vi "Read Interval.vi"(8 "error in (no error)":errorcluster, 11 "CS++PVMonitor in":refnum<class "CS++PVMonitor.lvclass">) -> (0 "error out":errorcluster, 2 "Interval":dbl[unit], 3 "CS++PVMonitor out":refnum<class "CS++PVMonitor.lvclass">)   [LabVIEW 2013, in "CS++PVMonitor.lvlib" / "CS++PVMonitor.lvclass"]
doc: "Read interval or timeout."
uses:
  CS++PVMonitor.lvclass
  CS++PVMonitor.lvclass/CS++PVMonitor.ctl
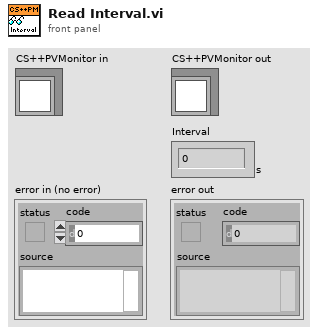
[diagram p1: front panel]
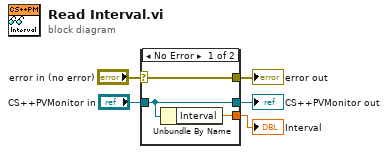
[diagram p0: block diagram]
diagram:
  n1 = case shown="No Error" "error in (no error)" {
    selector: "error in (no error)" -> [w8 w9]
    tunnel: [w8 w9] -> w4
    tunnel: [w7 w10] -> w2
    tunnel: "CS++PVMonitor in" -> [w7 w10]
    tunnel: [w6 _] -> w1
    frame No Error {
      n2 = Unbundle By Name(w7) -> ("Interval"=w6:dbl[unit])
    }
    frame Error {
    }
  }
  "error out" <- w4
  "CS++PVMonitor out" <- w2
  "Interval" <- w1
